vi "Create Timer Handler.vi"(8 "error in (no error)":errorcluster, 11 "Timer Index":u32) -> (0 "error out":errorcluster, 2 "Event Registration Refnum":refnum<event-registration>, 3 "Timer Handler":T1)   [LabVIEW 2024]
doc: "Creates a timer handler, including a timer index and user-defined events. These user-defined events include a start event, a stop event and an exit event."
uses:
  Timer Handler.ctl
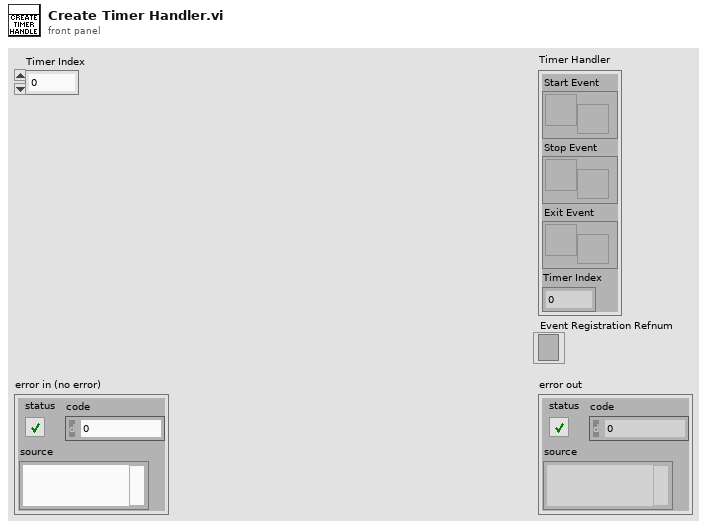
[diagram p1: front panel]
types:
  T1 = typedef "Timer Handler.ctl" = cluster{"Start Event":refnum<user-event>, "Stop Event":refnum<user-event>, "Exit Event":refnum<user-event>, "Timer Index":u32}
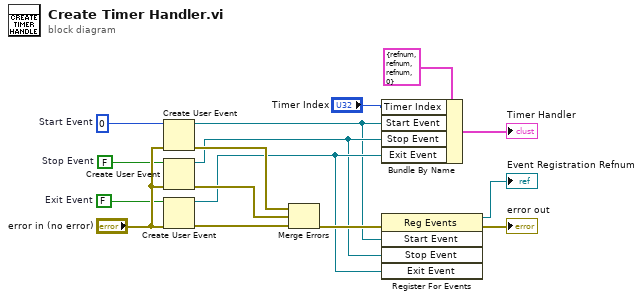
[diagram p0: block diagram]
diagram:
  w1 = u32 0  # Start Event
  w6 = FALSE  # Exit Event
  w7 = FALSE  # Stop Event
  n1 = Create User Event(user event datatype=w1, error in="error in (no error)") -> (user event=w2:refnum<user-event>, error out=w10:errorcluster)
  n2 = Create User Event(user event datatype=w7, error in="error in (no error)") -> (user event=w3:refnum<user-event>, error out=w9:errorcluster)
  n3 = Create User Event(user event datatype=w6, error in="error in (no error)") -> (user event=w4:refnum<user-event>, error out=w8:errorcluster)
  n4 = Merge Errors(w10, w9, w8) -> (w5:errorcluster)
  n5 = Bundle By Name(cluster=T1 {"Start Event"=refnum, "Stop Event"=refnum, "Exit Event"=refnum, "Timer Index"=0}, "Timer Index"="Timer Index", "Start Event"=w2, "Stop Event"=w3, "Exit Event"=w4) -> (→"Timer Handler":T1)
  n6 = register-events(error in=w5, w2, w3, w4) -> (reference out=→"Event Registration Refnum":refnum<event-registration>, error out=→"error out":errorcluster)  [unwired: 1 in]
